vi "mydaqMarcoGonzalez.vi"() -> ()   [LabVIEW 2012]
panel:
  in  "Array":bool[](array[boolean])
  in  "stop":bool
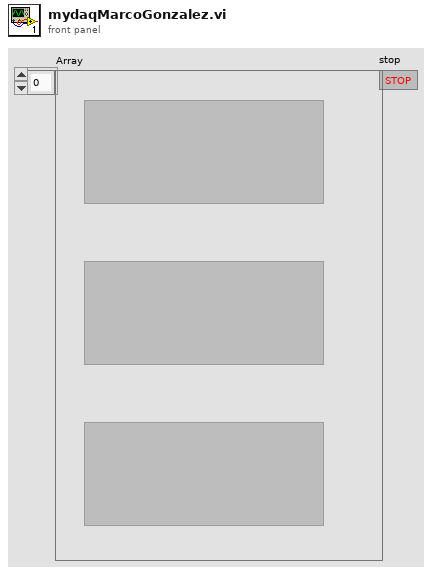
[diagram p1: front panel]
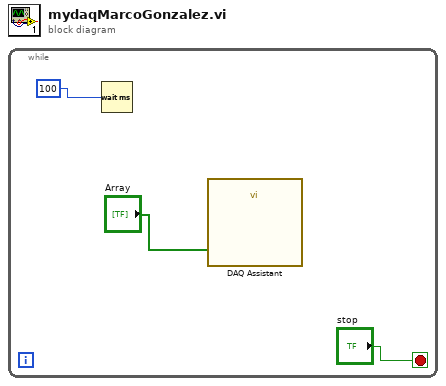
[diagram p0: block diagram]
diagram:
  n1 = while {
    stop <- "stop" stop-if-true
    n2 = Wait (ms)(milliseconds to wait=100) -> ()  [unwired: 1 out]
    n3 = call "DAQ Assistant"("data"="Array") -> ()  [unwired: 17 in, 2 out]
  }
